vi "WAIT_FOR_PID_RESET.vi"(10 "argv":string[](array[string]), 11 "args":u8) -> ()   [LabVIEW 2015]
uses:
  Team Code/Robot Global Data.vi
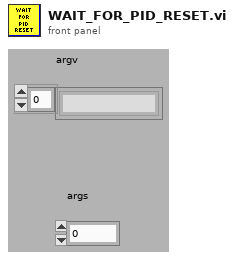
[diagram p1: front panel]
types:
  T1 = enum16{"ResetForward", "ResetBack", "PIDControl", "ManualControl", "ZeroEncoderAndTarget", "AutoStack"}
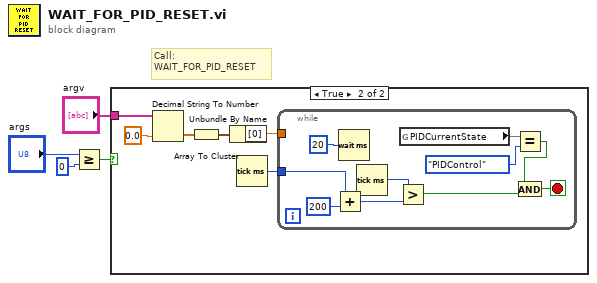
[diagram p0: block diagram]
diagram:
  # "Call:\nWAIT_FOR_PID_RESET"
  n1 = Greater Or Equal?(x="args", y=u8 0) -> (x >= y?=w4:bool)
  n2 = case shown="True" w4 {
    tunnel: "argv" -> [_ w10]
    frame False {
    }
    frame True {
      n3 = Decimal String To Number(string=w10, default (0L)=0.0 ("default (0 I32)")) -> (number=w8:dbl[])  [unwired: 2 out]
      n4 = Array To Cluster(array=w8) -> (cluster=w7:cluster{"[0]":dbl, "[1]":dbl})
      n5 = Unbundle By Name(w7) -> ("[0]"=w6:dbl)
      n6 = Tick Count (ms)() -> (millisecond timer value=w5:u32)
      n7 = while {
        tunnel: w6 -> [_]
        tunnel: w5 -> [w15]
        stop <- w12 stop-if-true
        n8 = Add(x=w15, y=u32 200) -> (x+y=w16:u32)
        n9 = Wait (ms)(milliseconds to wait=u32 20 ("millisecond multiple")) -> ()  [unwired: 1 out]
        n10 = Tick Count (ms)() -> (millisecond timer value=w17:u32)
        n11 = Greater?(x=w17, y=w16) -> (0:w11:bool)
        n12 = global read "Robot Global Data.vi" "PIDCurrentState"() -> (w18)
        n13 = Equal?(x=w18, y=T1."PIDControl") -> (x = y?=w13:bool)
        n14 = And(x=w13, y=w11) -> (x .and. y?=w12:bool)
      }
    }
  }
